vi "Meas Generate File Name.vi"(5 "waveforms folder":string="RAW", 7 "measurement header file name":string="session.info", 9 "meas id":i32, 10 "name base":string, 11 "folder":path) -> (0 "raw measurement data folder (MATs)":path, 1 "header file full path":path, 2 "measurement root folder":path, 3 "measurement full name":string, 4 "waveforms folder out":string="RAW")   [LabVIEW 2020]
doc: "Generates full measurement file name base. It takes 'name base' and replaces following variables in the name base:\n%id% - 'meas id' in format DDDD\n%date% - current date in format YYYYMMDD\n%time% - current time in format HH-MM-SS\n\nIt also returns combined full path with folder path."
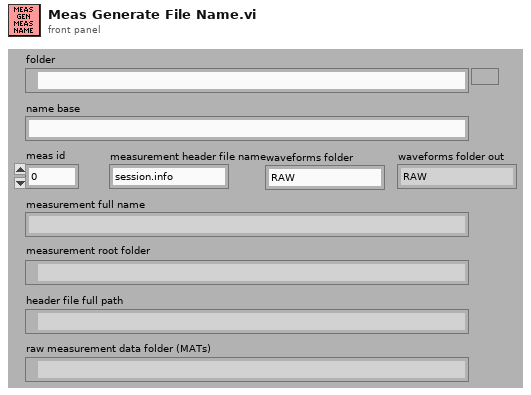
[diagram p1: front panel]
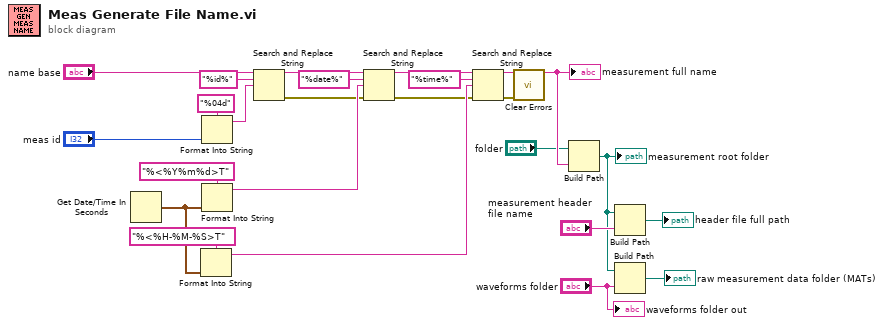
[diagram p0: block diagram]
diagram:
  n1 = Get Date/Time In Seconds() -> (seconds since 1Jan1904=w15:timestamp)
  n2 = Format Into String(format string="%<%H-%M-%S>T", w15) -> (resulting string=w11:string)  [unwired: 2 in, 1 out]
  n3 = Format Into String(format string="%04d", "meas id") -> (resulting string=w21:string)  [unwired: 2 in, 1 out]
  n4 = Format Into String(format string="%<%Y%m%d>T", w15) -> (resulting string=w16:string)  [unwired: 2 in, 1 out]
  n5 = Search and Replace String(input string="name base", search string="%id%", replace string=w21) -> (result string=w19:string, error out=w10:errorcluster)  [unwired: 5 in, 2 out]
  n6 = Search and Replace String(input string=w19, search string="%date%", replace string=w16, error in=w10) -> (result string=w12:string, error out=w9:errorcluster)  [unwired: 4 in, 2 out]
  n7 = Search and Replace String(input string=w12, search string="%time%", replace string=w11, error in=w9) -> (result string=w8:string, error out=w6:errorcluster)  [unwired: 4 in, 2 out]
  "measurement full name" <- w8
  n8 = call <vilib>:"Clear Errors.vi"("error in (no error)"=w6) -> ()  [unwired: 5 in, 2 out]
  n9 = Build Path(base path="folder", name or relative path=w8) -> (appended path=w3:path)
  "measurement root folder" <- w3
  n10 = Build Path(base path=w3, name or relative path="measurement header file name") -> (appended path=→"header file full path":path)
  n11 = Build Path(base path=w3, name or relative path="waveforms folder") -> (appended path=→"raw measurement data folder (MATs)":path)
  "waveforms folder out" <- "waveforms folder"
